vi "Get_CWparameters.vi"(8 "error in (no error)":errorcluster, 9 "Active Channel":string, 11 "resource name":refnum<k15>) -> (0 "error out":errorcluster, 2 "output cluster":T1, 3 "reference out":refnum<k15>)   [LabVIEW 2015, in "MyToolsFunction.lvlib"]
uses:
  ICcamera/MyToolsFunction.lvlib
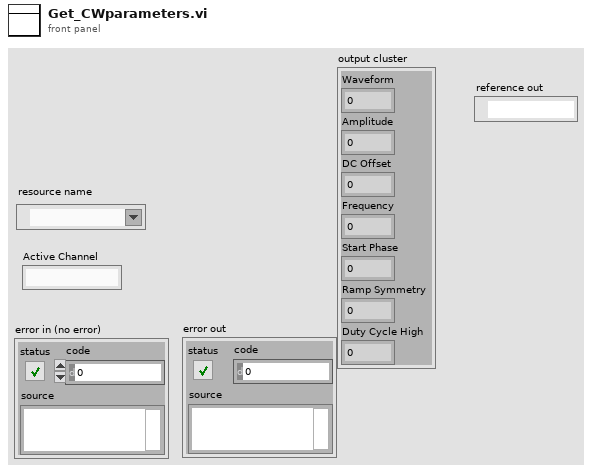
[diagram p1: front panel]
types:
  T1 = cluster{"Waveform":i32, "Amplitude":dbl, "DC Offset":dbl, "Frequency":dbl, "Start Phase":dbl, "Ramp Symmetry":dbl, "Duty Cycle High":dbl}
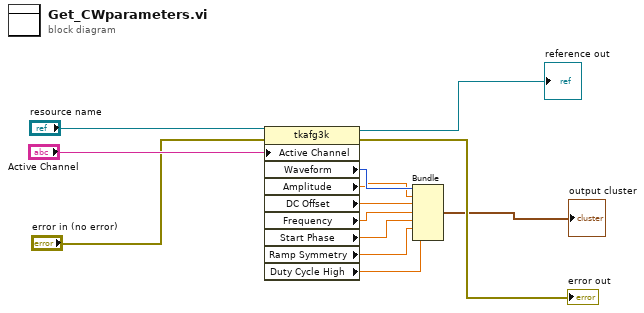
[diagram p0: block diagram]
diagram:
  n1 = property class="tkafg3k"(reference="resource name", error in="error in (no error)", "Active Channel"="Active Channel") -> (reference out=→"reference out":refnum<k15>, error out=→"error out":errorcluster, "Waveform"=w9:i32, "Amplitude"=w8:dbl, "DC Offset"=w7:dbl, "Frequency"=w6:dbl, "Start Phase"=w5:dbl, "Ramp Symmetry"=w4:dbl, "Duty Cycle High"=w3:dbl)
  n2 = Bundle("Waveform"=w9, "Amplitude"=w8, "DC Offset"=w7, "Frequency"=w6, "Start Phase"=w5, "Ramp Symmetry"=w4, "Duty Cycle High"=w3) -> (→"output cluster":T1)  [unwired: 1 in]
